vi "Read Timer.vi"(8 "error in (no error)":errorcluster, 11 "Timer in":refnum<class "Timer.lvclass">) -> (0 "error out":errorcluster, 1 "Time?Pulse":bool, 2 "Time?":bool, 3 "Timer out":refnum<class "Timer.lvclass">, 5 "Run":u32)   [LabVIEW 2011, in "Timer.lvclass"]
uses:
  Timer.lvclass
  Timer.lvclass/Timer.ctl
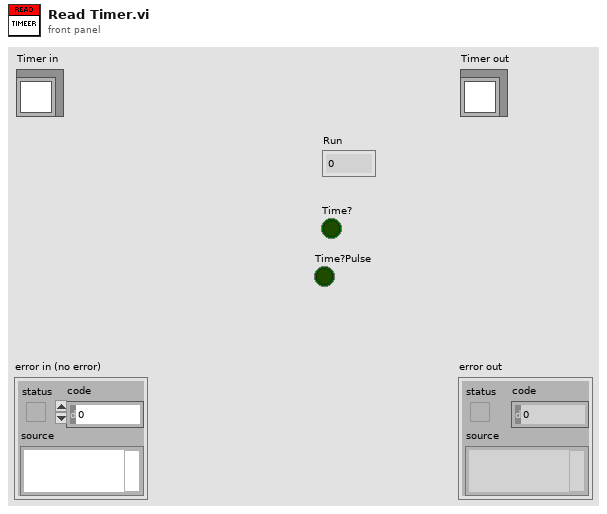
[diagram p1: front panel]
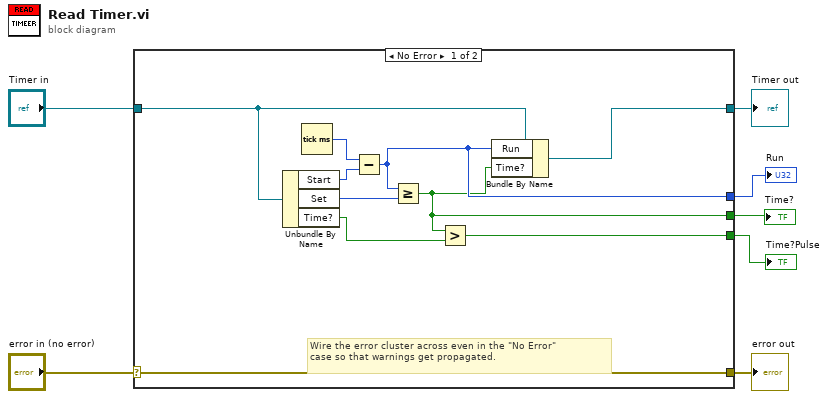
[diagram p0: block diagram]
diagram:
  n1 = case shown="No Error" "error in (no error)" {
    selector: "error in (no error)" -> [w17 w19]
    tunnel: [w17 w19] -> w6
    tunnel: [w12 w18] -> w4
    tunnel: "Timer in" -> [w13 w18]
    tunnel: [w11 _] -> w3
    tunnel: [w10 _] -> w2
    tunnel: [w8 _] -> w1
    frame No Error {
      # "Wire the error cluster across even in the \"No Error\"\ncase so that warnings get propagated."
      n2 = Unbundle By Name(w13) -> ("Start"=w15:u32, "Set"=w14:u32, "Time?"=w9:bool)
      n3 = Tick Count (ms)() -> (millisecond timer value=w16:u32)
      n4 = Subtract(x=w16, y=w15) -> (x-y=w11:u32)
      n5 = Greater Or Equal?(x=w11, y=w14) -> (x >= y?=w10:bool)
      n6 = Greater?(x=w10, y=w9) -> (0:w8:bool)
      n7 = Bundle By Name(cluster=w13, "Run"=w11, "Time?"=w10) -> (w12:refnum<class "Timer.lvclass">)
    }
    frame Error {
    }
  }
  "error out" <- w6
  "Timer out" <- w4
  "Run" <- w3
  "Time?" <- w2
  "Time?Pulse" <- w1
